vi "Read VISA resource.vi"(8 "error in (no error)":errorcluster, 11 "VISA Instrument in":refnum<class "VISA Instrument.lvclass">) -> (0 "error out":errorcluster, 2 "VISA resource":refnum<visa-resource-name>, 3 "VISA Instrument out":refnum<class "VISA Instrument.lvclass">)   [LabVIEW 2015, in "VISA Instrument.lvclass"]
uses:
  VISA Instrument.lvclass
  VISA Instrument.lvclass/VISA Instrument.ctl
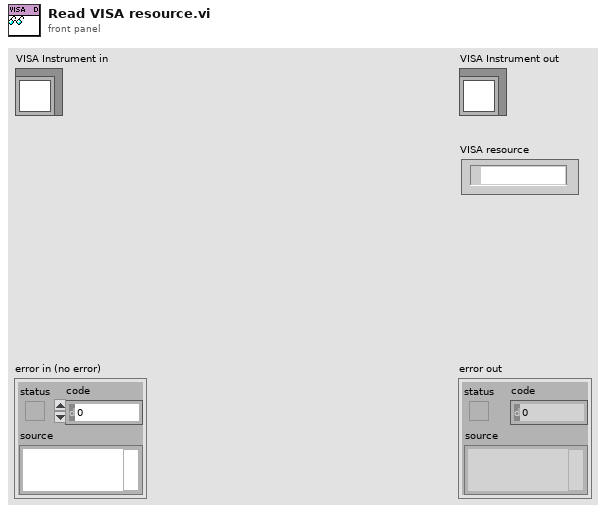
[diagram p1: front panel]
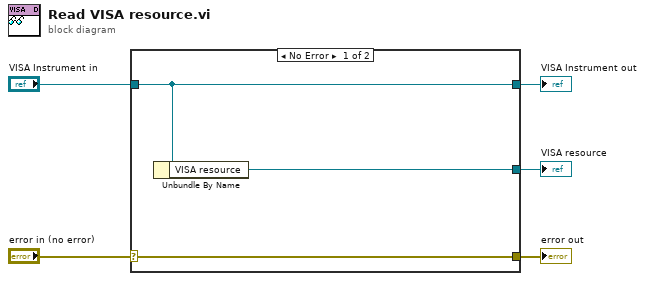
[diagram p0: block diagram]
diagram:
  n1 = case shown="No Error" "error in (no error)" {
    selector: "error in (no error)" -> [w8 w9]
    tunnel: [w8 w9] -> w4
    tunnel: [w7 w10] -> w2
    tunnel: "VISA Instrument in" -> [w7 w10]
    tunnel: [w6 _] -> w1
    frame No Error {
      n2 = Unbundle By Name(w7) -> ("VISA resource"=w6:refnum<visa-resource-name>)
    }
    frame Error {
    }
  }
  "error out" <- w4
  "VISA Instrument out" <- w2
  "VISA resource" <- w1
